vi "Parse_mFETmCAP_DmFET.vi"(0 "mFET_reply":string="0xDF10,pH,03/21/2017 20:36:40,0,-1.00,-1.0000,-1.0000,33,0,0,25.46,40.46,11.684,5.080e-02,7.0527,20.476,3.65,-0.985058,0.000029,-0.927686,0.000174,-1.225734,0.000054,+1.000e+00,-1.343e-08\r\n") -> (10 "Reply to save":string[](array[string])=["03/16/2017 02:10:49", "15", "24.04", "44.29", "11.788", "3.597", "+0.022770", "0.000035", "-1.611893", "0.000036", "+1.000e+00", "-1.000e+00"], 11 "Ib":dbl, 13 "Ik":dbl, 14 "float_array":dbl[](array[numeric]), 16 "Vrs_ext":dbl, 17 "Vrs_ext std":dbl, 18 "Vk":dbl, 19 "Vk std":dbl)   [LabVIEW 2022 SP3]
panel:
  out "Humidity_cont":dbl
  out "TC_Controller":dbl
  out "BiasBatt- V":dbl
  out "BiasBatt+ V":dbl
  out "MainBatt V":dbl
  out "SampleNum":dbl
  out "Datetime_cont":dbl
  out "Ib":string
  out "Ik":string
  out "Vk_std":string
  out "Vk":string="-1.000e+00"
  out "Vrs_ext_std":string="+1.000e+00"
  out "Vrs_ext":string="0.000036"
  out "Full Data Transmission?":bool
  # "Vtherm"
  # "Vtherm_std"
  # "TC"
  # "Vrse"
  # "Vrse_std"
  # "Vk"
  # "Vk_std"
  # "Ik"
  # "Ib"
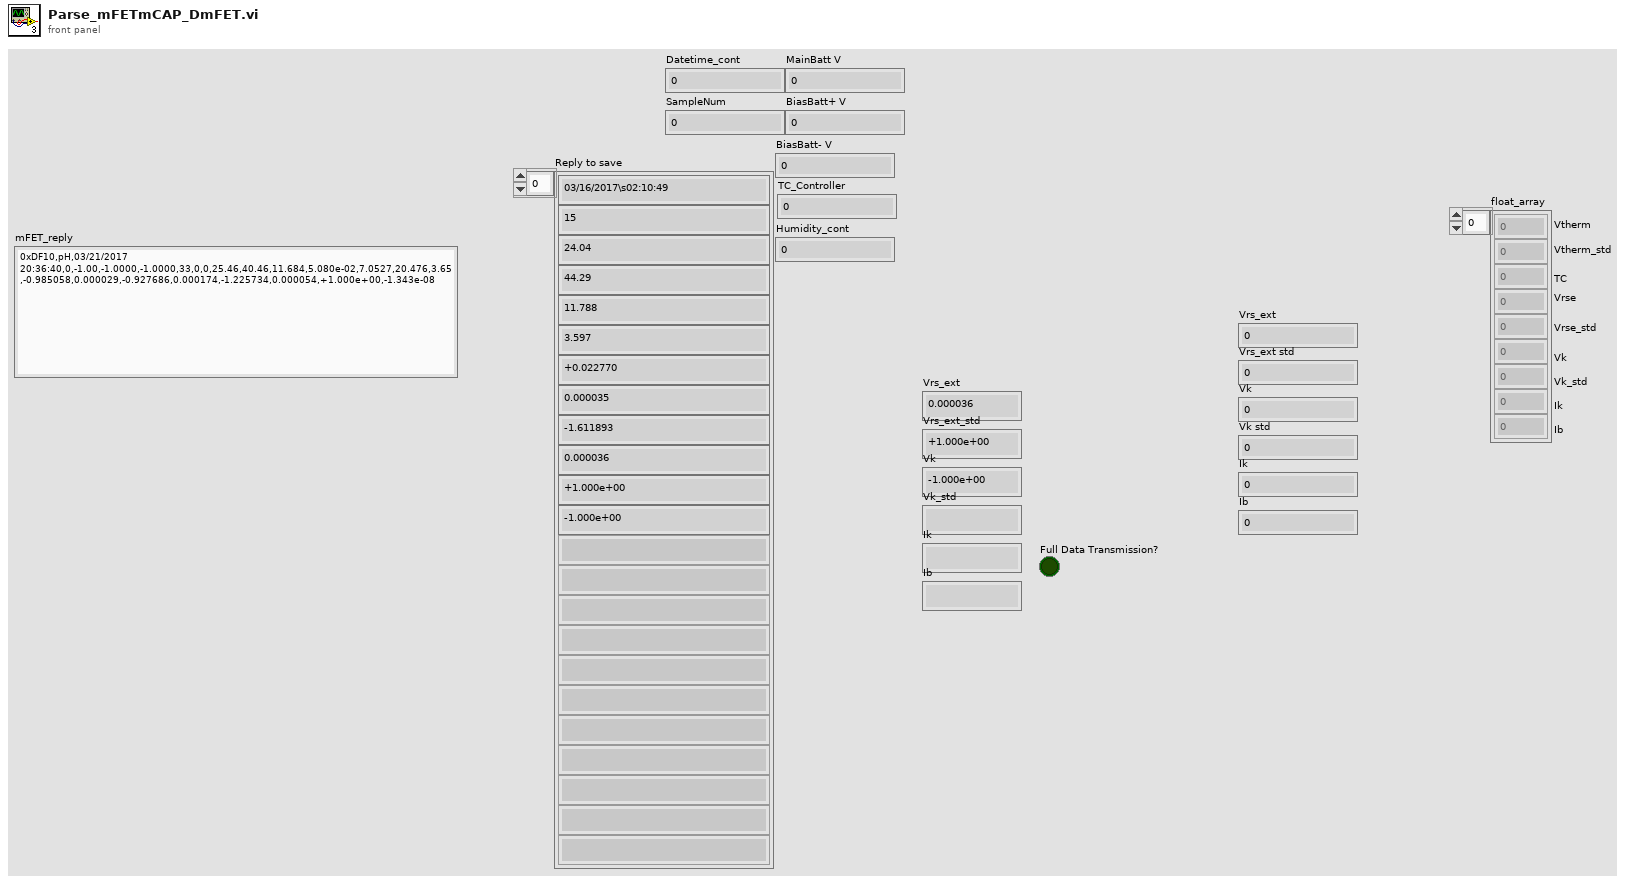
[diagram p1: front panel]
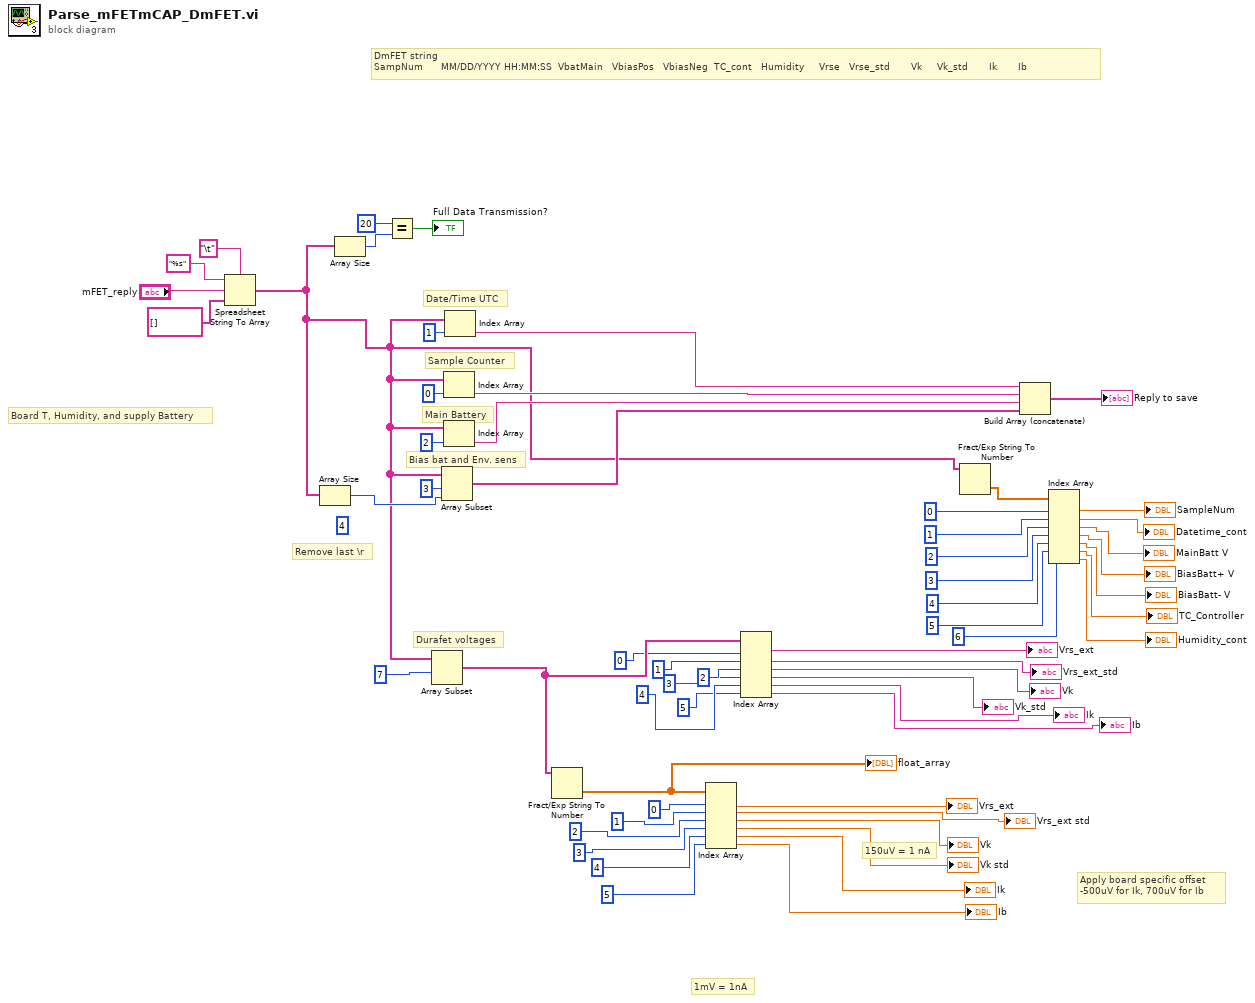
[diagram p0: block diagram]
diagram:
  (unwired) 4 ("y")
  # "DmFET string\nSampNum\t     MM/DD/YYYY HH:MM:SS\t VbatMain\t  VbiasPos\t  VbiasNeg\t TC_cont\t  Humidity\t    Vrse\t  Vrse_std\t      Vk\t    Vk_std\t      Ik\t      Ib"
  # "Remove last \\r"
  # "Bias bat and Env. sens"
  # "Main Battery"
  # "150uV = 1 nA"
  # "1mV = 1nA"
  # "Apply board specific offset \n-500uV for Ik, 700uV for Ib"
  # "Durafet voltages"
  # "Board T, Humidity, and supply Battery"
  # "Sample Counter"
  # "Date/Time UTC"
  n1 = Spreadsheet String To Array(delimiter (Tab)="\t", format string="%s", spreadsheet string="mFET_reply", array type (2D Dbl)=string[] []) -> (array=w16:string[])
  n2 = Array Size(array=w16) -> (size(s)=w41:i32)
  n3 = Array Size(array=w16) -> (size(s)=w52:i32)
  n4 = Equal?(x=20, y=w52) -> (x = y?=→"Full Data Transmission?":bool)
  n5 = Array Subset(array=w16, index=7) -> (w44:string[])  [unwired: 1 in]
  n6 = Array Subset(array=w16, index=3, length=w41) -> (w43:string[])
  n7 = Index Array(array=w16, index=0) -> (element=w48:string)
  n8 = Index Array(array=w16, index=2) -> (element=w42:string)
  n9 = Index Array(array=w16, index=1) -> (element=w49:string)
  n10 = Fract/Exp String To Number(string=w44) -> (number=w46:dbl[])  [unwired: 3 in, 1 out]
  "float_array" <- w46
  n11 = Index Array(array=w46, index #1=0 ("index"), index #2=1 ("index"), index #3=2 ("index"), index #4=3 ("index"), index #5=4 ("index"), index #6=5 ("index")) -> (element #1=→"Vrs_ext":dbl, element #2=→"Vrs_ext std":dbl, element #3=→"Vk":dbl, element #4=→"Vk std":dbl, element #5=→"Ik":dbl, element #6=→"Ib":dbl)
  n12 = Index Array(array=w44, index #1=0 ("index"), index #2=1 ("index"), index #3=2 ("index"), index #4=3 ("index"), index #5=4 ("index"), index #6=5 ("index")) -> (element #1=→"Vrs_ext":string, element #2=→"Vrs_ext_std":string, element #3=→"Vk":string, element #4=→"Vk_std":string, element #5=→"Ik":string, element #6=→"Ib":string)
  n13 = Fract/Exp String To Number(string=w16) -> (number=w15:dbl[])  [unwired: 3 in, 1 out]
  n14 = Build Array (concatenate)(w49, w48, w42, w43) -> (→"Reply to save":string[])
  n15 = Index Array(array=w15, index #1=0 ("index"), index #2=1 ("index"), index #3=2 ("index"), index #4=3 ("index"), index #5=4 ("index"), index #6=5 ("index"), index #7=6 ("index")) -> (element #1=→"SampleNum":dbl, element #2=→"Datetime_cont":dbl, element #3=→"MainBatt V":dbl, element #4=→"BiasBatt+ V":dbl, element #5=→"BiasBatt- V":dbl, element #6=→"TC_Controller":dbl, element #7=→"Humidity_cont":dbl)
